vi "Find Child UIDs.vi"(11 "TEMPLATE Actor in":refnum<class "TEMPLATE Actor.lvclass">) -> (2 "Child UIDs":T1)   [LabVIEW 2025, in "_Template.lvlib" / "Templates.lvlib" / "TEMPLATE Actor.lvlib" / "TEMPLATE Actor.lvlib" / "TEMPLATE Actor.lvclass"]
uses:
  TEMPLATE Actor.lvclass
  jettl/jettl/Child UIDs.ctl
  jettl/jettl/Actor/Actor.lvclass
  TEMPLATE Actor.lvclass/TEMPLATE Actor.ctl
  jettl/jettl/jettl.lvlib
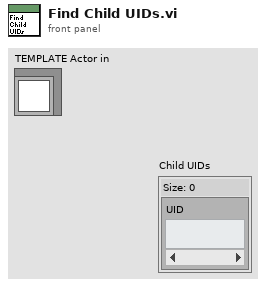
[diagram p1: front panel]
types:
  T1 = typedef "jettl.lvlib/Child UIDs.ctl" = set{string}
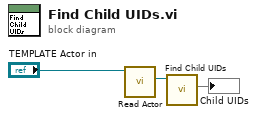
[diagram p0: block diagram]
diagram:
  n1 = call-dynamic "Read Actor.vi"("TEMPLATE Actor in"="TEMPLATE Actor in") -> ("Actor"=w1:refnum<class "Actor.lvclass">)  [unwired: 10 in]
  n2 = call-dynamic "Find Child UIDs.vi"("Actor in"=w1) -> ("Child UIDs"=→"Child UIDs":T1)  [unwired: 10 in]
